vi "PowerX 2D SGL.vi"(8 "Multiplier":sgl, 9 "Divider":sgl=100.0, 10 "Power":sgl, 11 "Signal In":sgl[][](array[numeric])) -> (3 "Signal Out":sgl[][](array[numeric]))   [LabVIEW 2023]
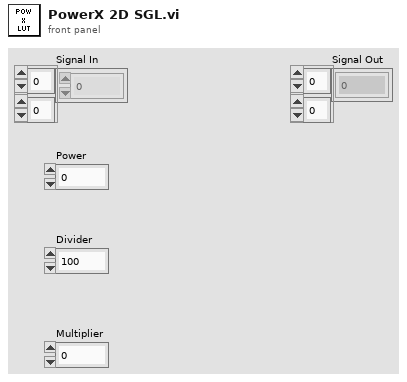
[diagram p1: front panel]
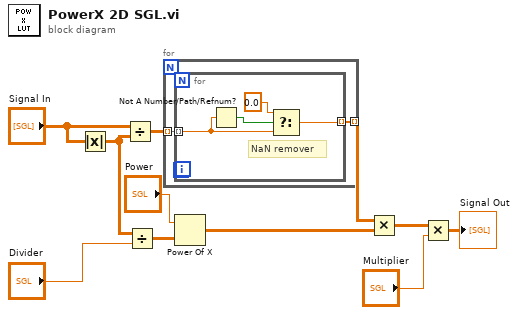
[diagram p0: block diagram]
diagram:
  n1 = Absolute Value(x="Signal In") -> (abs(x)=w1:sgl[][])
  n2 = Divide(x="Signal In", y=w1) -> (x/y=w3:sgl[][])
  n3 = Divide(x=w1, y="Divider") -> (x/y=w5:sgl[][])
  n4 = for {
    tunnel: [w13] -> w4 mode=indexing
    tunnel: w3 -> [w12] mode=indexing
    n5 = for {
      tunnel: w12 -> [w15] mode=indexing
      tunnel: [w16] -> w13 mode=indexing
      # "NaN remover"
      n6 = Not A Number/Path/Refnum?(number/path/refnum=w15) -> (NaN/Path/Refnum?=w14:bool)
      n7 = Select(t=sgl 0.0, s=w14, f=w15) -> (s? t:f=w16:sgl)
    }
  }
  n8 = Power Of X(1:w5, 2:"Power") -> (0:w6:sgl[][])
  n9 = Multiply(x=w4, y=w6) -> (x*y=w2:sgl[][])
  n10 = Multiply(x=w2, y="Multiplier") -> (x*y=→"Signal Out":sgl[][])
